vi "solar_log Menu.vi"(5 "MenuRef (Activation only)":refnum<k9>, 7 "ItemTag (Selection only)":string, 8 "error in (no error)":errorcluster, 9 "Coords":T1, 10 "ListBox in":refnum<vi>) -> (0 "error out":errorcluster)   [LabVIEW 2018]
doc: "This activates and handles the right-click menu options for the logger status listbox. Place this VI in the <b>Listbox : Shortcut Menu Activation?</b> and <b>Listbox : Shortcut Menu Selection (User)</b> event cases."
uses:
  <vilib>/Utility/error.llb/DialogType.ctl
  <vilib>/Utility/miscctls.llb/LVPoint32TypeDef.ctl
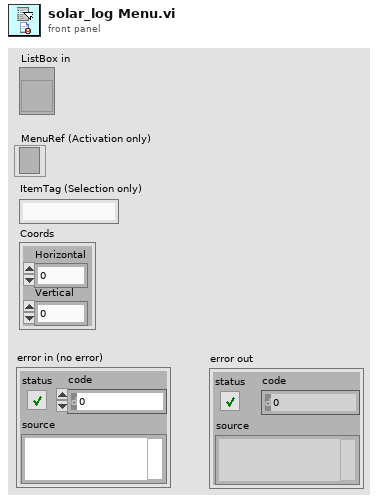
[diagram p1: front panel]
types:
  T1 = typedef "LVPoint32TypeDef.ctl" = cluster{"Horizontal":i32, "Vertical":i32}
  T2 = typedef "DialogType.ctl" = u16
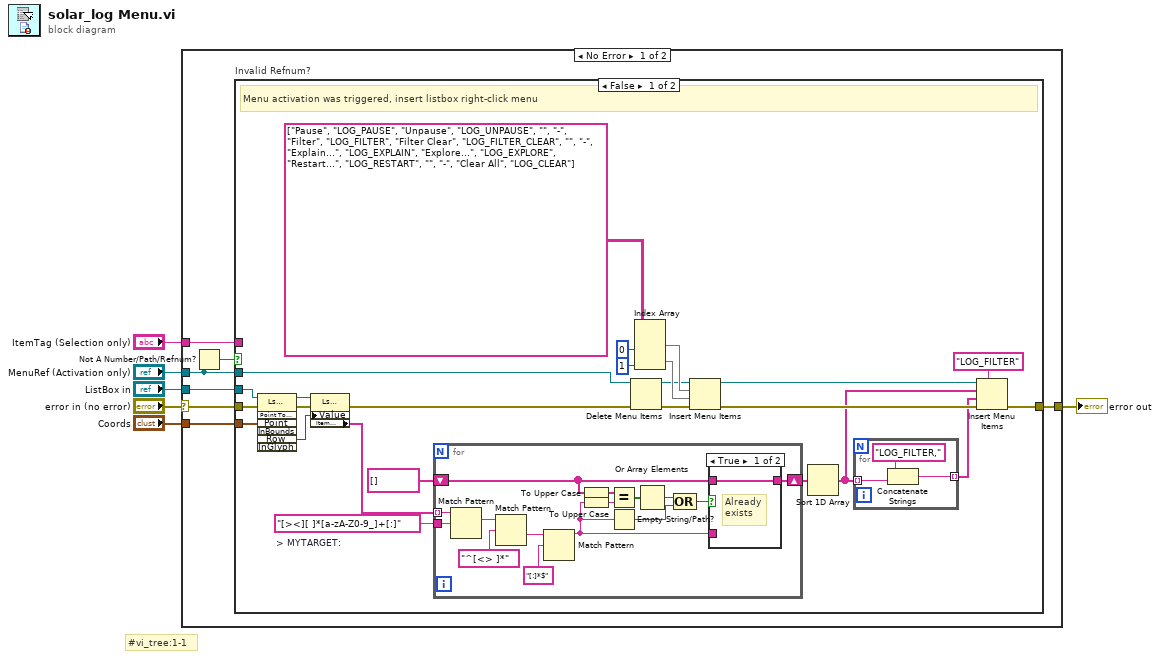
[diagram p0: block diagram]
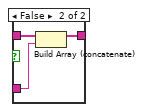
[diagram p2: hidden frame]
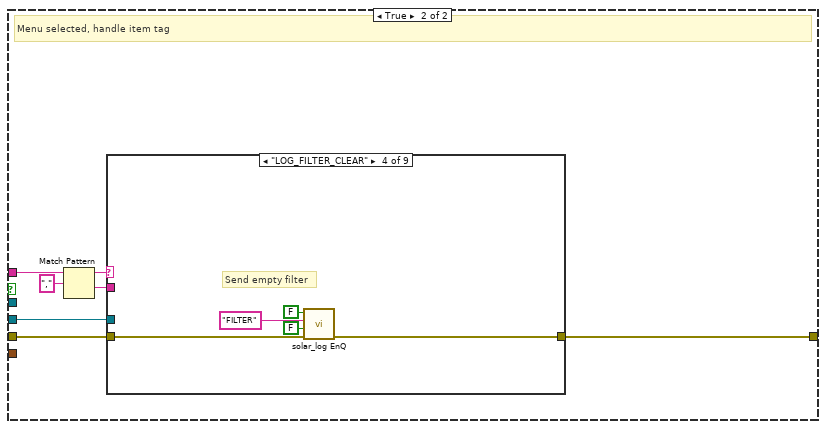
[diagram p3: hidden frame]
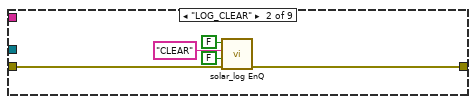
[diagram p5: hidden frame]
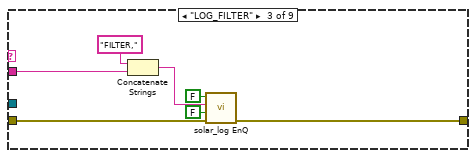
[diagram p6: hidden frame]
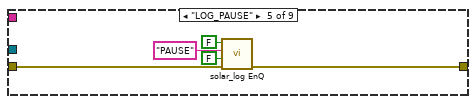
[diagram p7: hidden frame]
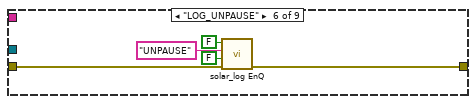
[diagram p8: hidden frame]
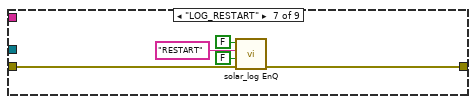
[diagram p9: hidden frame]
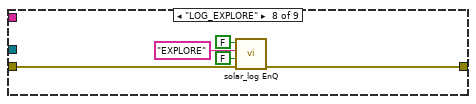
[diagram p10: hidden frame]
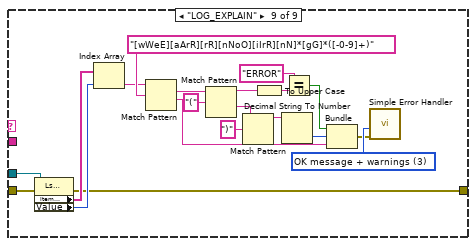
[diagram p11: hidden frame]
diagram:
  # "#vi_tree:1-1"
  n1 = case shown="No Error" "error in (no error)" {
    selector: "error in (no error)" -> [w11 w126]
    tunnel: "Coords" -> [w13 _]
    tunnel: "ListBox in" -> [w12 _]
    tunnel: [w10 w126] -> w3
    tunnel: "MenuRef (Activation only)" -> [w9 _]
    tunnel: "ItemTag (Selection only)" -> [w7 _]
    frame No Error {
      n2 = Not A Number/Path/Refnum?(number/path/refnum=w9) -> (NaN/Path/Refnum?=w8:bool)
      n3 = case "Invalid Refnum?" shown="False" w8 {
        tunnel: w13 -> [w35 _]
        tunnel: w12 -> [w34 w66]
        tunnel: w9 -> [w27 _]
        tunnel: w11 -> [w26 w67]
        tunnel: [w16 w65] -> w10
        tunnel: w7 -> [_ w64]
        frame False {
          w23 = "[><][ ]*[a-zA-Z0-9_]+[:]"  # > MYTARGET:
          # "Menu activation was triggered, insert listbox right-click menu"
          n4 = invoke class="LstBox (strict)" method="Point To Row"(reference=w34, error in=w26, "Point"=w35) -> (reference out=w36:refnum<vi>, error out=w37:errorcluster, "Row"=w24:i32)  [unwired: 4 in, 4 out]
          n5 = property class="LstBox (strict)"(reference=w36, error in=w37, "Value"=w24) -> (error out=w38:errorcluster, "Item Names"=w22:string[])  [unwired: 1 out]
          n6 = for {
            tunnel: w23 -> [w56]
            tunnel: w22 -> [w51] mode=indexing
            shift-right: [w50] -> w17
            shift-left: string[] [] -> [w49]
            n7 = Match Pattern(string=w51, regular expression=w56) -> (match substring=w55:string)  [unwired: 1 in, 3 out]
            n8 = Match Pattern(string=w55, regular expression="^[<> ]*") -> (after substring=w53:string)  [unwired: 1 in, 3 out]
            n9 = Match Pattern(string=w53, regular expression="[:]*$") -> (before substring=w44:string)  [unwired: 1 in, 3 out]
            n10 = To Upper Case(1:w49) -> (0:w48:string[])
            n11 = To Upper Case(1:w44) -> (0:w47:string)
            n12 = Equal?(x=w48, y=w47) -> (x = y?=w46:bool[])
            n13 = Empty String/Path?(string/path=w44) -> (empty?=w43:bool)
            n14 = Or Array Elements(Boolean array=w46) -> (logical OR=w45:bool)
            n15 = Compound Arithmetic op=OR(w45, w43) -> (w42:bool)
            n16 = case shown="True" w42 {
              tunnel: [w57 w59] -> w50
              tunnel: w49 -> [w57 w60]
              tunnel: w44 -> [_ w58]
              frame True {
                # "Already\nexists"
              }
              frame False {
                n17 = Build Array (concatenate)(w60, w58) -> (w59:string[])
              }
            }
          }
          n18 = Delete Menu Items(6:w38, 9:w27) -> (0:w29:errorcluster, 3:w28:refnum<k9>)  [unwired: 2 in]
          n19 = Index Array(array=string[][] [["Pause", "LOG_PAUSE"], ["Unpause", "LOG_UNPAUSE"], ["", "-"], ["Filter", "LOG_FILTER"], ["Filter Clear", "LOG_FILTER_CLEAR"], ["", "-"], ["Explain...", "LOG_EXPLAIN"], ["Explore...", "LOG_EXPLORE"], ["Restart...", "LOG_RESTART"], ["", "-"], ["Clear All", "LOG_CLEAR"]], index (col) #1=0 ("disabled index (col)"), index (col) #2=1 ("index (col)")) -> (element #1=w32:string[], element #2=w33:string[])  [unwired: 2 in]
          n20 = Insert Menu Items(6:w29, 7:w33, 8:w32, 9:w28) -> (0:w21:errorcluster, 3:w20:refnum<k9>)  [unwired: 2 in, 1 out]
          n21 = Sort 1D Array(array=w17) -> (sorted array=w15:string[])
          n22 = for {
            tunnel: w15 -> [w40] mode=indexing
            tunnel: [w39] -> w14 mode=indexing
            n23 = Concatenate Strings("LOG_FILTER,", w40) -> (w39:string)
          }
          n24 = Insert Menu Items(5:"LOG_FILTER" ("menu tag"), 6:w21, 7:w14, 8:w15, 9:w20) -> (0:w16:errorcluster)  [unwired: 1 in, 2 out]
        }
        frame True {
          # "Menu selected, handle item tag"
          n25 = Match Pattern(string=w64, regular expression=",") -> (before substring=w63:string, after substring=w61:string)  [unwired: 1 in, 2 out]
          n26 = case shown="\"LOG_FILTER_CLEAR\"" w63 {
            tunnel: w66 -> [_ _ _ _ _ _ _ _ w125]
            tunnel: w67 -> [w68 w70 w77 w83 w87 w92 w96 w101 w107]
            tunnel: [w68 w69 w76 w82 w86 w91 w97 w102 w106] -> w65
            tunnel: w61 -> [_ _ w74 _ _ _ _ _ _]
            frame Default {
            }
            frame "LOG_CLEAR" {
              n27 = call "solar_log EnQ.vi"("error in (no error)"=w70, "Front? (F)"=FALSE, "MSG"="CLEAR", "Create? (F)"=FALSE) -> ("error out"=w69:errorcluster)  [unwired: 5 in, 2 out]
            }
            frame "LOG_FILTER" {
              n28 = Concatenate Strings("FILTER," ("MSG"), w74) -> (w75:string)
              n29 = call "solar_log EnQ.vi"("error in (no error)"=w77, "Front? (F)"=FALSE, "MSG"=w75, "Create? (F)"=FALSE) -> ("error out"=w76:errorcluster)  [unwired: 5 in, 2 out]
            }
            frame "LOG_FILTER_CLEAR" {
              # "Send empty filter"
              n30 = call "solar_log EnQ.vi"("error in (no error)"=w83, "Front? (F)"=FALSE, "MSG"="FILTER", "Create? (F)"=FALSE) -> ("error out"=w82:errorcluster)  [unwired: 5 in, 2 out]
            }
            frame "LOG_PAUSE" {
              n31 = call "solar_log EnQ.vi"("error in (no error)"=w87, "Front? (F)"=FALSE, "MSG"="PAUSE", "Create? (F)"=FALSE) -> ("error out"=w86:errorcluster)  [unwired: 5 in, 2 out]
            }
            frame "LOG_UNPAUSE" {
              n32 = call "solar_log EnQ.vi"("error in (no error)"=w92, "Front? (F)"=FALSE, "MSG"="UNPAUSE", "Create? (F)"=FALSE) -> ("error out"=w91:errorcluster)  [unwired: 5 in, 2 out]
            }
            frame "LOG_RESTART" {
              n33 = call "solar_log EnQ.vi"("error in (no error)"=w96, "Front? (F)"=FALSE, "MSG"="RESTART", "Create? (F)"=FALSE) -> ("error out"=w97:errorcluster)  [unwired: 5 in, 2 out]
            }
            frame "LOG_EXPLORE" {
              n34 = call "solar_log EnQ.vi"("error in (no error)"=w101, "Front? (F)"=FALSE, "MSG"="EXPLORE", "Create? (F)"=FALSE) -> ("error out"=w102:errorcluster)  [unwired: 5 in, 2 out]
            }
            frame "LOG_EXPLAIN" {
              w124 = T2 3 items=["no dialog", "OK message", "continue or stop message", "OK message + warnings", "continue/stop + warnings"] ("type of dialog (OK msg:1)")
              n35 = property class="LstBox (strict)"(reference=w125, error in=w107) -> (error out=w106:errorcluster, "Item Names"=w109:string[], "Value"=w108:i32)  [unwired: 1 out]
              n36 = Index Array(array=w109, index=w108) -> (element=w122:string)
              n37 = Match Pattern(string=w122, regular expression="[wWeE][aArR][rR][nNoO][iIrR][nN]*[gG]*([-0-9]+)") -> (match substring=w121:string, after substring=w111:string)  [unwired: 1 in, 2 out]
              n38 = Match Pattern(string=w121, regular expression="(") -> (before substring=w116:string, after substring=w118:string)  [unwired: 1 in, 2 out]
              n39 = Match Pattern(string=w118, regular expression=")") -> (before substring=w117:string)  [unwired: 1 in, 3 out]
              n40 = To Upper Case(1:w116) -> (0:w114:string)
              n41 = Decimal String To Number(string=w117) -> (number=w112:i32)  [unwired: 2 in, 1 out]
              n42 = Equal?(x="ERROR", y=w114) -> (x = y?=w113:bool)
              n43 = Bundle(w113, w112, w111) -> (w110:errorcluster)  [unwired: 1 in]
              n44 = call <vilib>:"Simple Error Handler.vi"("type of dialog (OK msg:1)"=w124, "error in (no error)"=w110) -> ()  [unwired: 3 in, 5 out]
            }
          }
        }
      }
    }
    frame Error {
    }
  }
  "error out" <- w3
